vi "4Pi Focus Lock - FFT shift 2D.vi"(11 "Input image":sgl[][](array[numeric])) -> (3 "fft shifted image":sgl[][](array[numeric]))   [LabVIEW 2016]
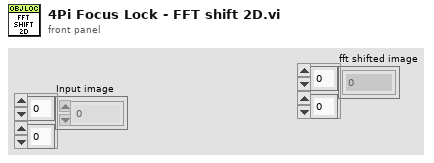
[diagram p1: front panel]
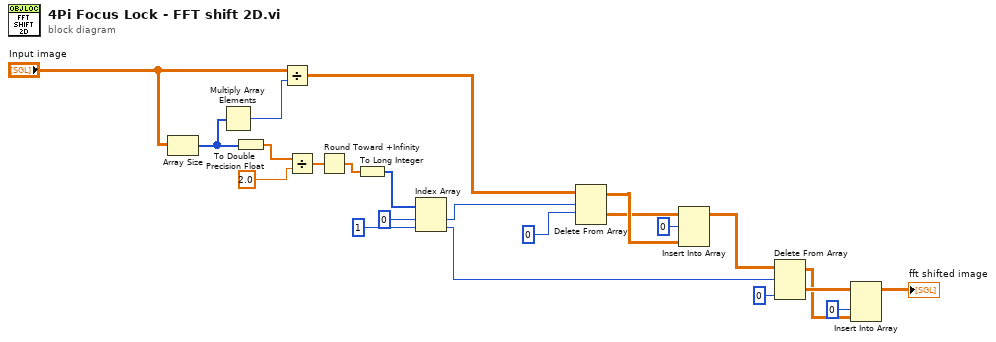
[diagram p0: block diagram]
diagram:
  n1 = Array Size(array="Input image") -> (size(s)=w20:i32[])
  n2 = Multiply Array Elements(1:w20) -> (0:w21:i32)
  n3 = To Double Precision Float(number=w20) -> (double precision float=w4:dbl[])
  n4 = Divide(x="Input image", y=w21) -> (x/y=w22:sgl[][])
  n5 = Divide(x=w4, y=2.0 ("index")) -> (x/y=w6:dbl[])
  n6 = Round Toward +Infinity(x=w6) -> (ceil(x): smallest int >= x=w7:dbl[])
  n7 = To Long Integer(number=w7) -> (32bit integer=w8:i32[])
  n8 = Index Array(array=w8, index #1=0 ("index"), index #2=1 ("index")) -> (element #1=w12:i32, element #2=w15:i32)
  n9 = Delete From Array(array=w22, length=w12, index (row)=0 ("index")) -> (deleted portion=w10:sgl[][], array with subset deleted=w11:sgl[][])  [unwired: 1 in]
  n10 = Insert Into Array(array=w10, index (row)=0, new element=w11) -> (w14:sgl[][])  [unwired: 1 in]
  n11 = Delete From Array(array=w14, length=w15, index (col)=0 ("disabled index (col)")) -> (deleted portion=w18:sgl[][], array with subset deleted=w17:sgl[][])  [unwired: 1 in]
  n12 = Insert Into Array(array=w18, index (col)=0 ("index (row)"), new element=w17) -> (→"fft shifted image":sgl[][])  [unwired: 1 in]
